vi "Write Map.vi"(8 "error in (no error)":errorcluster, 10 "Map":T1, 11 "Remap Bus in":refnum<class "Alias Bus.lvclass">) -> (0 "error out":errorcluster, 3 "Remap Bus out":refnum<class "Alias Bus.lvclass">)   [LabVIEW 2021, in "Alias Bus.lvclass"]
uses:
  Alias Bus.lvclass
  Support/Remap Type.ctl
  Alias Bus.lvclass/Alias Bus.ctl
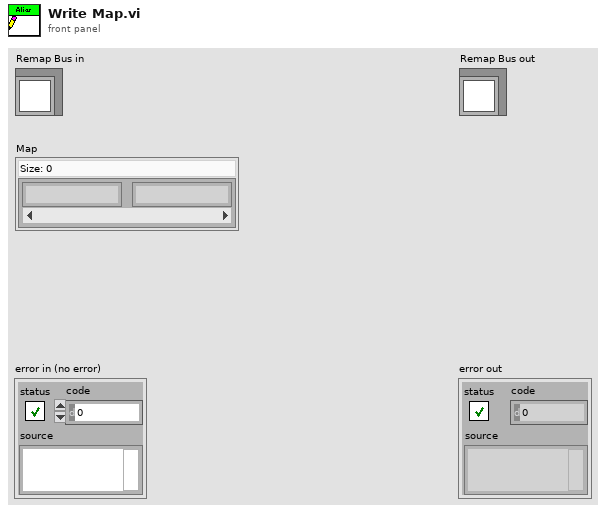
[diagram p1: front panel]
types:
  T1 = typedef "Alias Bus.lvclass/Remap Type.ctl" = map{string, string}
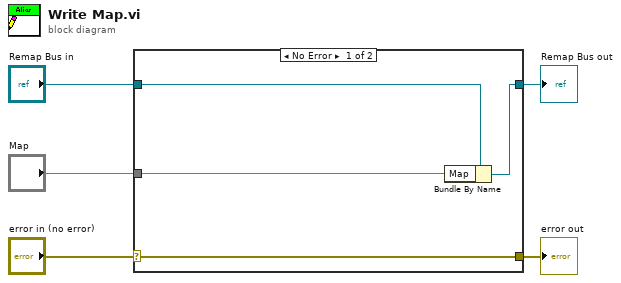
[diagram p0: block diagram]
diagram:
  n1 = case shown="No Error" "error in (no error)" {
    selector: "error in (no error)" -> [w9 w10]
    tunnel: [w9 w10] -> w4
    tunnel: [w7 w11] -> w2
    tunnel: "Remap Bus in" -> [w8 w11]
    tunnel: "Map" -> [w6 _]
    frame No Error {
      n2 = Bundle By Name(cluster=w8, "Map"=w6) -> (w7:refnum<class "Alias Bus.lvclass">)
    }
    frame Error {
    }
  }
  "error out" <- w4
  "Remap Bus out" <- w2
